vi "2dMatToNx1Mat.vi"(11 "2D Array":dbl[][](array[numeric])) -> (3 "nx1 Array":dbl[][](array[numeric]))   [LabVIEW 2016]
doc: "Transform mxn array to (m*n)x1 array."
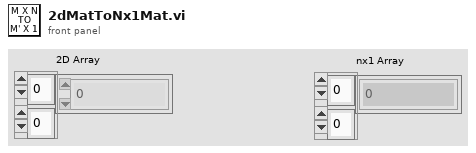
[diagram p1: front panel]
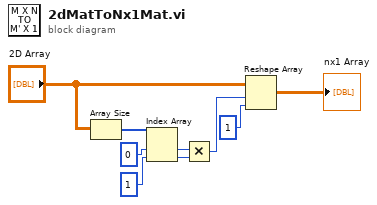
[diagram p0: block diagram]
diagram:
  n1 = Array Size(array="2D Array") -> (size(s)=w9:i32[])
  n2 = Index Array(array=w9, index #1=0 ("index"), index #2=1 ("index")) -> (element #1=w6:i32, element #2=w5:i32)
  n3 = Multiply(x=w6, y=w5) -> (x*y=w4:i32)
  n4 = Reshape Array("2D Array", w4, 1 ("dimension size")) -> (→"nx1 Array":dbl[][])
